vi "FUN_EC_ES (SubVI).vi"(6 "Den":dbl[](array[numeric]), 7 "Retardo(T)":dbl, 9 "Num":dbl[](array[numeric]), 10 "U(t)":dbl, 11 "d(t)":dbl) -> (0 "error out":errorcluster, 2 "y(t)":dbl format="%.2f", 3 "Función de transferencia.":T1)   [LabVIEW 2020]
uses:
  <vilib>/Analysis/baseanly.llb/Real Dot Product.vi
  <vilib>/Analysis/baseanly.llb/A x Vector.vi
  <vilib>/Analysis/NI_AALBase.lvlib
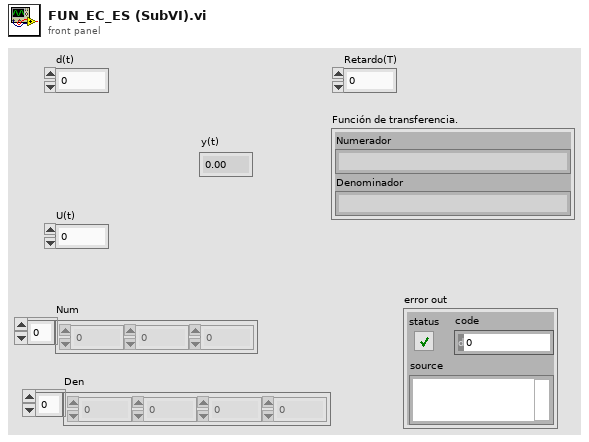
[diagram p1: front panel]
types:
  T1 = cluster{"Numerador":string, "Denominador":string}
  T2 = typedef "NI_Matrix.lvlib/RealMatrix.ctl" = dbl[][]
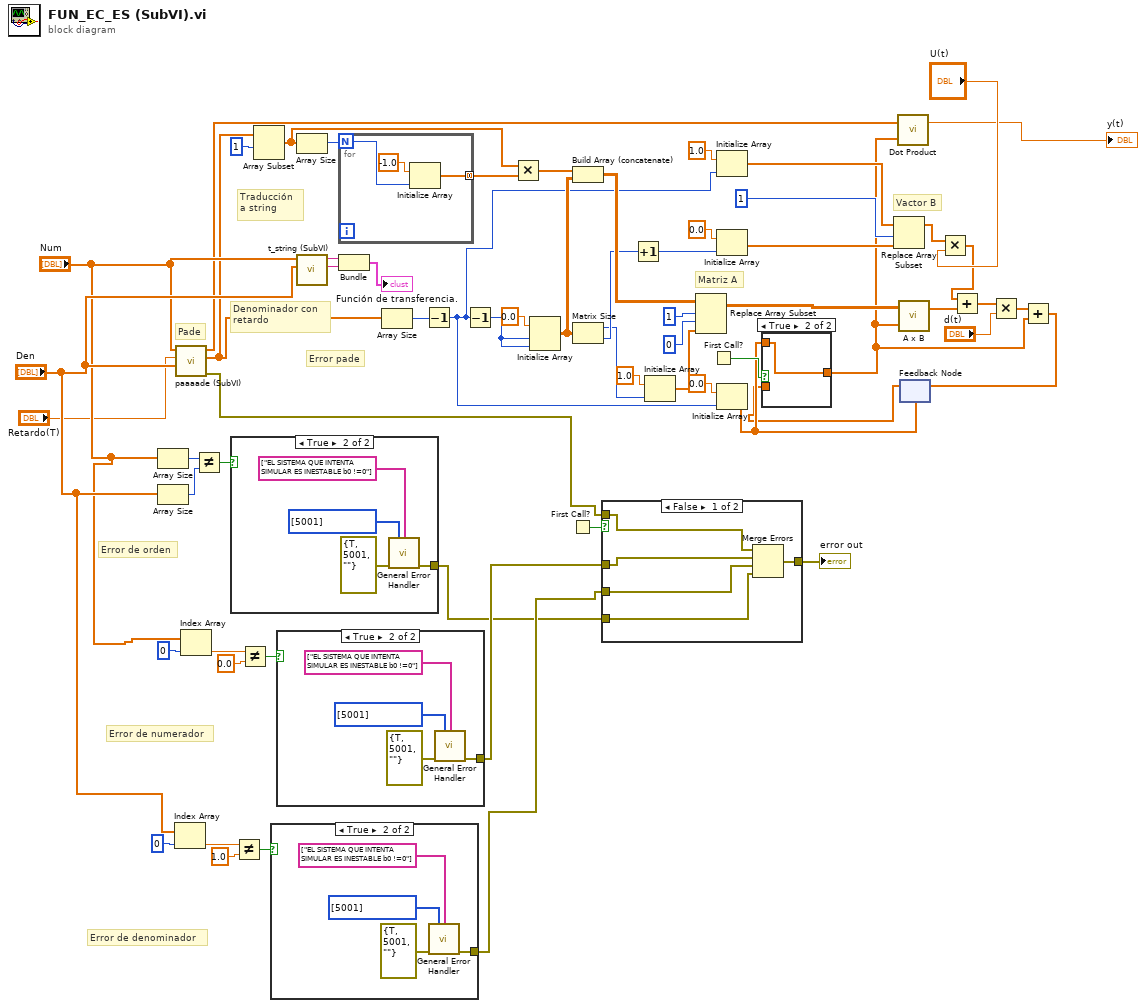
[diagram p0: block diagram]
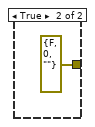
[diagram p3: hidden frame]
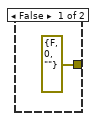
[diagram p4: hidden frame]
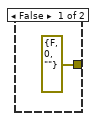
[diagram p5: hidden frame]
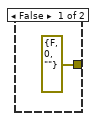
[diagram p6: hidden frame]
diagram:
  # "Error de denominador"
  # "Error de numerador"
  # "Error de orden"
  # "Error pade"
  # "Traducción \na string"
  # "Denominador con\nretardo"
  # "Vactor B"
  # "Matriz A"
  # "Pade"
  n1 = Array Size(array="Num") -> (size(s)=w52:i32)
  n2 = Array Size(array="Den") -> (size(s)=w53:i32)
  n3 = Index Array(array="Den", index=0) -> (element=w49:dbl)
  n4 = call "paaaade (SubVI).vi"("Den"="Den", "Retardo(T)"="Retardo(T)", "Num"="Num") -> ("error out"=w56:errorcluster, "Den_retard"=w12:dbl[], "Num_retard"=w38:dbl[])  [unwired: 6 in]
  n5 = Index Array(array="Num", index=0) -> (element=w45:dbl)
  n6 = Not Equal?(x=w52, y=w53) -> (x != y?=w51:bool)
  n7 = case shown="True" w51 {
    tunnel: [errorcluster {"status"=FALSE, "code"=0, "source"=""} ("error constant") w65] -> w57
    frame False {
    }
    frame True {
      n8 = call <vilib>:"General Error Handler.vi"("[user-defined codes]"=i32[] [5001], "[user-defined descriptions]"=string[] ["EL SISTEMA QUE INTENTA SIMULAR ES INESTABLE b0 !=0"], "error in (no error)"=errorcluster {"status"=TRUE, "code"=5001, "source"=""}) -> ("error out"=w65:errorcluster)  [unwired: 8 in, 4 out]
    }
  }
  n9 = Not Equal?(x=w49, y=1.0) -> (x != y?=w47:bool)
  n10 = Not Equal?(x=w45, y=0.0) -> (x != y?=w44:bool)
  n11 = Array Subset(array=w12, index=1) -> (w14:dbl[])  [unwired: 1 in]
  n12 = case shown="True" w47 {
    tunnel: [errorcluster {"status"=FALSE, "code"=0, "source"=""} ("error constant") w70] -> w59
    frame False {
    }
    frame True {
      n13 = call <vilib>:"General Error Handler.vi"("[user-defined codes]"=i32[] [5001], "[user-defined descriptions]"=string[] ["EL SISTEMA QUE INTENTA SIMULAR ES INESTABLE b0 !=0"], "error in (no error)"=errorcluster {"status"=TRUE, "code"=5001, "source"=""}) -> ("error out"=w70:errorcluster)  [unwired: 8 in, 4 out]
    }
  }
  n14 = case shown="True" w44 {
    tunnel: [errorcluster {"status"=FALSE, "code"=0, "source"=""} ("error constant") w75] -> w58
    frame False {
    }
    frame True {
      n15 = call <vilib>:"General Error Handler.vi"("[user-defined codes]"=i32[] [5001], "[user-defined descriptions]"=string[] ["EL SISTEMA QUE INTENTA SIMULAR ES INESTABLE b0 !=0"], "error in (no error)"=errorcluster {"status"=TRUE, "code"=5001, "source"=""}) -> ("error out"=w75:errorcluster)  [unwired: 8 in, 4 out]
    }
  }
  n16 = Array Size(array=w14) -> (size(s)=w13:i32)
  n17 = call "t_string (SubVI).vi"("Denominador"="Den", "Numerador"="Num") -> ("String"=w41:string, "String 2"=w40:string)  [unwired: 8 in]
  n18 = for {
    N: w13 -> [w81]
    tunnel: [w79] -> w15 mode=concatenating
    n19 = Initialize Array(-1.0 ("element"), w81) -> (w79:dbl[])
  }
  n20 = Bundle("String 2"=w40, "String"=w41) -> (→"Función de transferencia.":cluster{"String 2":string, "String":string})  [unwired: 1 in]
  n21 = Array Size(array=w12) -> (size(s)=w2:i32)
  n22 = Decrement(x=w2) -> (x-1=w1:i32)
  n23 = Decrement(x=w1) -> (x-1=w16:i32)
  n24 = Multiply(x=w14, y=w15) -> (x*y=w23:dbl[])
  n25 = Initialize Array(0.0 ("element"), w16, w16) -> (w22:dbl[][])
  n26 = First Call?() -> (First Call?: T/F=w54:bool)
  n27 = Build Array (concatenate)(w23, w22) -> (w28:T2)
  n28 = Matrix Size(0:w22) -> (1:w18:i32, 2:w19:i32)
  n29 = case shown="False" w54 {
    tunnel: [w86 errorcluster {"status"=FALSE, "code"=0, "source"=""} ("error constant")] -> w55
    tunnel: w56 -> [w85 _]
    tunnel: w57 -> [w84 _]
    tunnel: w58 -> [w83 _]
    tunnel: w59 -> [w82 _]
    frame False {
      n30 = Merge Errors(w85, w83, w82, w84) -> (w86:errorcluster)
    }
    frame True {
    }
  }
  "error out" <- w55
  n31 = Increment(x=w19) -> (x+1=w20:i32)
  n32 = Initialize Array(1.0 ("element"), w18) -> (w32:dbl[])
  n33 = Replace Array Subset(array=w28, new element=w32, index (row)=1 ("disabled index (row)"), index (col)=0 ("disabled index (col)")) -> (w4:T2)
  n34 = First Call?() -> (First Call?: T/F=w7:bool)
  n35 = Initialize Array(1.0 ("element"), w1) -> (w25:dbl[])
  n36 = Initialize Array(0.0 ("element"), w20) -> (w27:dbl[])
  n37 = Initialize Array(0.0 ("element"), w1) -> (w6:dbl[])
  n38 = Replace Array Subset(array=w25, new element=w27, index=1) -> (w9:dbl[])
  n39 = feedback #1(w6) -> (w5:dbl[])
  n40 = case shown="True" w7 {
    tunnel: w6 -> [_ w89]
    tunnel: w5 -> [w88 _]
    tunnel: [w88 w89] -> w3
    frame False {
    }
    frame True {
    }
  }
  n41 = call-poly <vilib>:"Dot Product.vi"("Y Vector"=w3, "X Vector"=w38) -> ("X * Y"=→"y(t)":dbl)  [unwired: 1 out]
  n42 = call-poly <vilib>:"A x B.vi"("Vector"=w3, "A"=w4) -> ("A x Vector"=w34:dbl[])  [unwired: 1 out]
  n43 = Multiply(x=w9, y="U(t)") -> (x*y=w8:dbl[])
  n44 = Add(x=w8, y=w34) -> (x+y=w35:dbl[])
  n45 = Multiply(x=w35, y="d(t)") -> (x*y=w36:dbl[])
  n46 = Add(x=w36, y=w3) -> (x+y=w37:dbl[])
  n47 = feedback-in #1(w37) -> ()
